vi "tm_closedcimgfile.vi"(8 "error in (no error)":errorcluster, 11 "File Handle":u32) -> (0 "error out":errorcluster)   [LabVIEW 2012]
uses:
  tmcamcon.dll
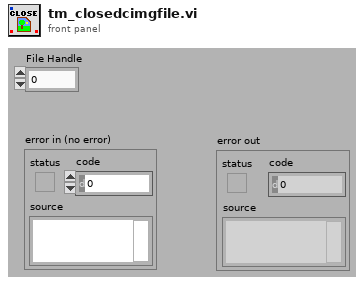
[diagram p1: front panel]
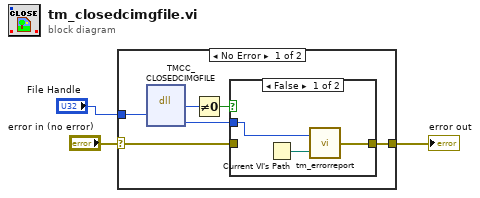
[diagram p0: block diagram]
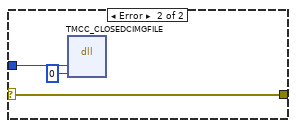
[diagram p3: hidden frame]
diagram:
  n1 = case shown="No Error" "error in (no error)" {
    selector: "error in (no error)" -> [w7 w16]
    tunnel: [w4 w16] -> w2
    tunnel: "File Handle" -> [w8 w15]
    frame No Error {
      n2 = dll-call lib="tmcamcon.dll" fn="TMCC_CLOSEDCIMGFILE"("filehandle"=w8) -> ("return type"=w9:u32, "Erval"=w6:i32)  [unwired: 5 in, 2 out]
      n3 = Not Equal To 0?(x=w9) -> (x != 0?=w5:bool)
      n4 = case shown="False" w5 {
        tunnel: w7 -> [_ w13]
        tunnel: [w11 w13] -> w4
        tunnel: w6 -> [w10 _]
        frame False {
          n5 = Current VI's Path() -> (path=w12:path)
          n6 = call "tm_errorreport.vi"("Source"=w12, "Error"=w10) -> ("error out"=w11:errorcluster)
        }
        frame True {
        }
      }
    }
    frame Error {
      n7 = dll-call lib="tmcamcon.dll" fn="TMCC_CLOSEDCIMGFILE"("filehandle"=w15, "Erval"=0) -> ()  [unwired: 6 in, 2 out]
    }
  }
  "error out" <- w2
